vi "I2C Write.vi"(1 "Min time SCL low (uSec)":u32, 2 "Min Time SCL high (uSec)":u32, 3 "Number of Bytes":i16, 4 "Data to send":u8[](array[numeric])) -> ()   [LabVIEW 2013]
uses:
  <vilib>/rvi/Emulation/niFpgaSctlEmulationGetInTimedLoop.vi
  <vilib>/rvi/Emulation/niFpgaEmulationReportErrorSimple.vi
  <vilib>/rvi/Emulation/niFpgaGetClockAttributes.vi
  <vilib>/rvi/eio/common/nirviEmuTemplateMethod_errors.vi
  <vilib>/rvi/Emulation/niFpgaCriticalErrorInLSC.vi
  <vilib>/eio/EIONode/EIONode.xnode
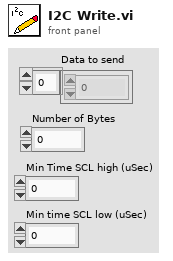
[diagram p1: front panel]
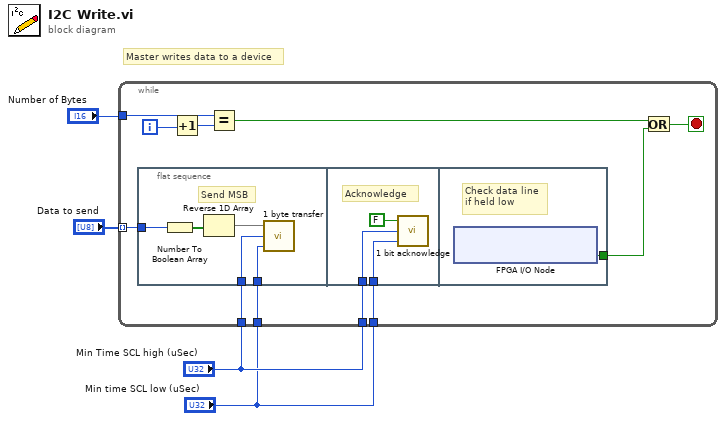
[diagram p0: block diagram]
diagram:
  # "Master writes data to a device"
  n1 = while {
    tunnel: "Number of Bytes" -> [w13]
    tunnel: "Min Time SCL high (uSec)" -> [w10]
    tunnel: "Min time SCL low (uSec)" -> [w9]
    tunnel: "Min Time SCL high (uSec)" -> [w8]
    tunnel: "Min time SCL low (uSec)" -> [w7]
    tunnel: "Data to send" -> [w6] mode=indexing
    i -> [w14]
    stop <- w12 stop-if-true
    n2 = flat-sequence {
      tunnel: w8 -> [w19]
      tunnel: w7 -> [w18]
      tunnel: w6 -> [w17]
      tunnel: w10 -> [w22]
      tunnel: w9 -> [w21]
      tunnel: [w24] -> w5
      frame #0 {
        # "Send MSB"
        n3 = Number To Boolean Array(number=w17) -> (Boolean array=w16:bool[])
        n4 = Reverse 1D Array(array=w16) -> (reversed array=w20:bool[])
        n5 = call "1 byte transfer.vi"("Min time SCL low (uSec)"=w18, "Min Time SCL high (uSec)"=w19, "Data bit array"=w20) -> ()  [unwired: 1 in]
      }
      frame #1 {
        # "Acknowledge"
        n6 = call "1 bit acknowledge.vi"("Min time SCL low (uSec)"=w21, "Min Time SCL high (uSec)"=w22, "Acknowledgement"=FALSE) -> ()  [unwired: 1 in]
      }
      frame #2 {
        # "Check data line\nif held low"
        n7 = xnode "FPGA I/O Node"() -> ("ConnectorB/DIO13"=w24:bool)  [unwired: 1 in, 1 out]
      }
    }
    n8 = Increment(x=w14) -> (x+1=w15:i32)
    n9 = Equal?(x=w13, y=w15) -> (x = y?=w11:bool)
    n10 = Or(x=w11, y=w5) -> (x .or. y?=w12:bool)
  }
